vi "Get.vi"(8 "error in":errorcluster) -> (0 "error out":errorcluster, 3 "Waveform In":waveform(dbl))   [LabVIEW 2020]
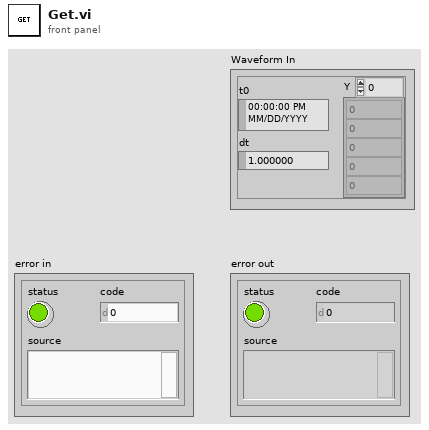
[diagram p1: front panel]
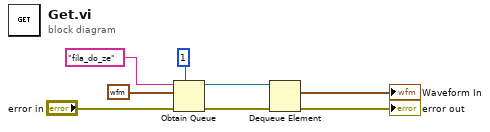
[diagram p0: block diagram]
diagram:
  n1 = Obtain Queue(max queue size (-1, unlimited)=1, name (unnamed)="fila_do_ze", element data type=waveform(dbl) {"t0"=timestamp(0 s since 1904-01-01), "dt"=1.0, "Y"=[]} ("Waveform"), error in (no error)="error in") -> (queue out=w6:refnum<queue>, error out=w5:errorcluster)  [unwired: 1 in, 1 out]
  n2 = Dequeue Element(queue=w6, error in (no error)=w5) -> (element=→"Waveform In":waveform(dbl), error out=→"error out":errorcluster)  [unwired: 1 in, 2 out]
